vi "数据列表.vi"() -> (3 "数组":T1(array[cluster]))   [LabVIEW 2016, in "DGUS.lvlib"]
uses:
  DGUS.lvlib
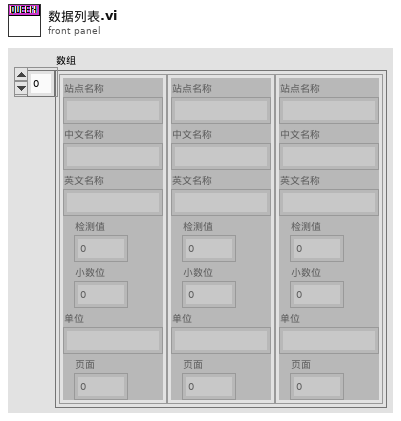
[diagram p1: front panel]
types:
  T1 = cluster{"站点名称":string, "中文名称":string, "英文名称":string, "检测值":sgl, "小数位":u8, "单位":string, "页面":u16}[]
  T2 = cluster{"站点名称":string, "中文名称":string, "英文名称":string, "检测值":sgl, "小数位":u8, "单位":string, "页面":u16}
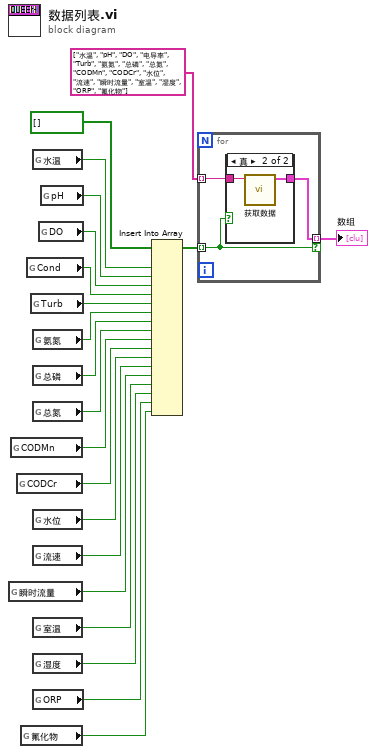
[diagram p0: block diagram]
diagram:
  n1 = global read "副屏设置全局变量.vi" "瞬时流量"() -> (w8:bool)
  n2 = global read "副屏设置全局变量.vi" "CODMn"() -> (w12:bool)
  n3 = global read "副屏设置全局变量.vi" "CODCr"() -> (w11:bool)
  n4 = global read "副屏设置全局变量.vi" "氟化物"() -> (w2:bool)
  n5 = global read "副屏设置全局变量.vi" "Cond"() -> (w17:bool)
  n6 = global read "副屏设置全局变量.vi" "Turb"() -> (w16:bool)
  n7 = global read "副屏设置全局变量.vi" "水温"() -> (w20:bool)
  n8 = global read "副屏设置全局变量.vi" "氨氮"() -> (w15:bool)
  n9 = global read "副屏设置全局变量.vi" "总磷"() -> (w14:bool)
  n10 = global read "副屏设置全局变量.vi" "总氮"() -> (w13:bool)
  n11 = global read "副屏设置全局变量.vi" "水位"() -> (w10:bool)
  n12 = global read "副屏设置全局变量.vi" "流速"() -> (w9:bool)
  n13 = global read "副屏设置全局变量.vi" "室温"() -> (w7:bool)
  n14 = global read "副屏设置全局变量.vi" "湿度"() -> (w6:bool)
  n15 = global read "副屏设置全局变量.vi" "ORP"() -> (w3:bool)
  n16 = global read "副屏设置全局变量.vi" "DO"() -> (w18:bool)
  n17 = global read "副屏设置全局变量.vi" "pH"() -> (w19:bool)
  n18 = Insert Into Array(array=bool[] [], new element #1=w20, new element #2=w19, new element #3=w18, new element #4=w17, new element #5=w16, new element #6=w15, new element #7=w14, new element #8=w13, new element #9=w12, new element #10=w11, new element #11=w10, new element #12=w9, new element #13=w8, new element #14=w7, new element #15=w6, new element #16=w3, new element #17=w2) -> (w5:bool[])  [unwired: 1 in]
  n19 = for {
    tunnel: w5 -> [w22] mode=indexing
    tunnel: string[] ["水温", "pH", "DO", "电导率", "Turb", "氨氮", "总磷", "总氮", "CODMn", "CODCr", "水位", "流速", "瞬时流量", "室温", "湿度", "ORP", "氟化物"] -> [w24] mode=indexing
    tunnel: [w23] -> w1 mode=indexing if=w22
    n20 = case shown="真" w22 {
      tunnel: w24 -> [_ w26]
      tunnel: [_ w25] -> w23
      frame False {
      }
      frame True {
        n21 = call "获取数据.vi"("table"=w26) -> ("输出簇"=w25:T2)  [unwired: 10 in]
      }
    }
  }
  "数组" <- w1
